vi "get_crystal_position.vi"(8 "error in":errorcluster, 10 "Crystal Number":u16(ring) items=["Crystal 1", "Crystal 2", "Crystal 3", "Crystal 4", "Crystal 5", "Crystal 6", "Crystal 7", ""], 11 "address":string) -> (0 "error out":errorcluster, 2 "Crystal Number Out":u16(ring) items=["Crystal 1", "Crystal 2", "Crystal 3", "Crystal 4", "Crystal 5", "Crystal 6", "Crystal 7", ""], 3 "Crystal Position":i32)   [LabVIEW 2020]
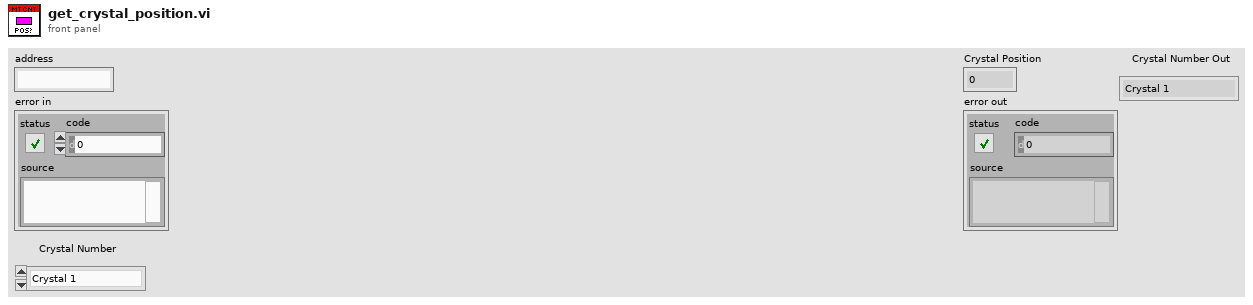
[diagram p1: front panel]
types:
  T1 = enum16{"Standard", "Buffered", "CRLF", "Immediate"}
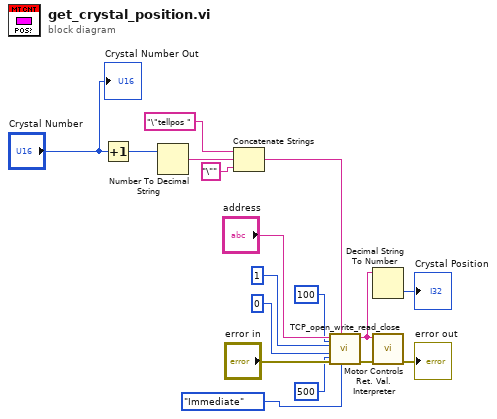
[diagram p0: block diagram]
diagram:
  n1 = Increment(x="Crystal Number") -> (x+1=w16:u16)
  n2 = Number To Decimal String(number=w16) -> (decimal integer string=w9:string)  [unwired: 1 in]
  n3 = Concatenate Strings("\"tellpos " ("write string"), w9, "\"" ("string")) -> (w7:string)
  n4 = call "TCP_open_write_read_close.vi"("timeout ms (25000)"=500, "bytes to read"=100, "mode (standard)"=T1."Immediate", "write string"=w7, "error in"="error in", "local port (0)"=u16 0, "remote port or service name"=u16 1, "address"="address") -> ("error out"=w4:errorcluster, "read string"=w2:string)  [unwired: 2 in]
  n5 = Decimal String To Number(string=w2) -> (number=→"Crystal Position":i32)  [unwired: 2 in, 1 out]
  n6 = call "Motor Controls Ret. Val. Interpreter.vi"("error in"=w4, "Command Return"=w2) -> ("error out"=→"error out":errorcluster)  [unwired: 8 in, 1 out]
  "Crystal Number Out" <- "Crystal Number"
